vi "On Open Document.vi"(0 "PDF Report IN":T23(xcontrol), 11 "error in (no error)":errorcluster) -> (4 "PDF Report OUT":T23(xcontrol), 15 "error out":errorcluster)   [LabVIEW 2013]
doc: "Developed by Jean-Marc Simard\nCopyright © 2010, Exaprom Inc.\nAll rights reserved.\nLicense: BSD\n\nWith iTextSharp 4.1.6 (http://itextsharp.sourceforge.net)\nunder Mozilla Public License Version 1.1\n(http://www.mozilla.org/MPL/MPL-1.1.html)"
uses:
  C:/Users/MaxCorp/Documents/GitHub/TopView/DLL/itextsharp.dll
  DLL/itextsharp.dll
  Controls/PDF Report Xcontrol/PDF Report.xctl
  Controls/Font size.ctl
  Controls/Font color.ctl
  Controls/Font cluster.ctl
  Controls/Header footer horiz alignment.ctl
  <userlib>/Exaprom PDF/Controls/Watermark Page Position.ctl
  Controls/Watermark cluster.ctl
panel:
  out "Font OUT":T1={"Name"="Helvetica", "Size"=12.0, "Color"=0, "Style"={"Bold"=FALSE, "Italic"=FALSE, "Underline"=FALSE, "Strikeout"=FALSE}}
  in  "Font IN":T1={"Name"="Helvetica", "Size"=12.0, "Color"=0, "Style"={"Bold"=FALSE, "Italic"=FALSE, "Underline"=FALSE, "Strikeout"=FALSE}}
  in  "input cluster":T4={"Show? (F)"=FALSE, "Watermark type"=enum."Text", "Opacity (%)"=0.0, "Alignment"=enum."Center", "Rotate(°)"=0.0, "Watermark"=enum."Absolute", "X (mm)"=5.0, "Y (mm)"=30.0, "Text"="JMS", "Font"={"Name"="", "Size"=12.0, "Color"=0, "Style"={"Bold"=FALSE, "Italic"=FALSE, "Underline"=FALSE, "Strikeout"=FALSE}}, "Image path"=path "", "Image (%)"=100.0}
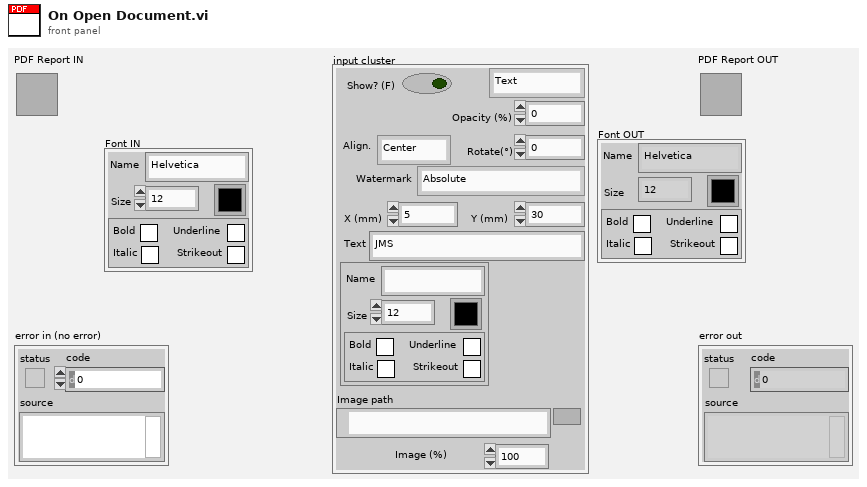
[diagram p1: front panel]
types:
  T1 = typedef "Font cluster.ctl" = cluster{"Name":string, "Size":T2, "Color":T3, "Style":cluster{"Bold":bool, "Italic":bool, "Underline":bool, "Strikeout":bool}}
  T2 = typedef "Font size.ctl" = sgl
  T3 = typedef "Font color.ctl" = u32
  T4 = typedef "Watermark cluster.ctl" = cluster{"Show? (F)":bool, "Watermark type":enum16{"Text", "Text auto", "Image"}, "Opacity (%)":sgl, "Alignment":T5, "Rotate(°)":sgl, "Watermark":T6, "X (mm)":sgl, "Y (mm)":sgl, "Text":string, "Font":T1, "Image path":path, "Image (%)":sgl}
  T5 = typedef "Header footer horiz alignment.ctl" = enum16{"Left", "Center", "Right"}
  T6 = typedef "Watermark Page Position.ctl" = enum16{"Absolute", "Center on page", "Center on text section"}
  T7 = typedef "Unit.ctl" = enum16{"inch", "mm"}
  T8 = typedef "Paragraphe cluster.ctl" = cluster{" Aligment":T9, "Line spacing":T10}
  T9 = typedef "Texte alignement.ctl" = enum16{"Select", "CENTER", "JUSTIFY", "LEFT", "RIGHT"}
  T10 = typedef "Line spacing.ctl" = enum16{"Select", "1.0", "1.5", "2.0"}
  T11 = typedef "Page dimensions.ctl" = cluster{"Start at page":i32, "Orientation":T12, "widht":sgl, "height":sgl, "Margin left":sgl, "Margin right":sgl, "Margin top":sgl, "Margin bottom":sgl}
  T12 = typedef "Page Orientation.ctl" = enum16{"Portrait", "Landscape"}
  T13 = typedef "Image or Table Caption.ctl" = cluster{"Caption":string, "Separator":string, "Position":enum16{"Above", "Below"}}
  T14 = typedef "Header Footer [ ].ctl" = T15[]
  T15 = typedef "Header Footer cluster.ctl" = cluster{"Start page":i32, "Type":T16, "Alignment":T5, "Vertical Alignement":T17, "Image (%)":sgl, "Page #":T18, "Text":string, "Path":string, "Font":T1, "Font refnum":refnum<k24>, "Line":cluster{"Line":T19, "Thickness (points)":sgl, "Colour":T3}}
  T16 = typedef "Header Footer Type.ctl" = enum16{"Select", "Text", "Text + hyperlink", "Page number", "Image", "Image + hyperlink"}
  T17 = typedef "Cell Vertical alignment.ctl" = enum16{"TOP", "MIDDLE", "BOTTOM"}
  T18 = typedef "Page number.ctl" = cluster{"Text 1":string, "Text 2":string, "Text 3":string}
  T19 = typedef "Header Footer Line.ctl" = enum16{"No line", "Horizontal line"}
  T20 = typedef "Watermark cluster2.ctl" = cluster{"Show? (F)":bool, "Type":enum16{"Image", "Text"}, "Opacity (%)":sgl, "Rotate(°)":sgl, "Position":cluster{"Position":T21, "X":sgl, "Y":sgl}, "Image path":path, "Scaled(%)":sgl, "Image refnum":refnum<k24>, "Text":string, "Font":cluster{"Name":string, "Size":T2, "Color":T3}, "Font refnum":refnum<k24>, "Alignment":T5, "Automatic":bool}
  T21 = typedef "Watermark Position.ctl" = enum16{"Absolute", "Center (page)", "Center (text section)"}
  T22 = typedef "System Fonts.ctl" = cluster{"Font name [ ]":string[], "Font and file names [ ]":cluster{"Font name":string, "File name":string}[]}
  T23 = cluster{"Document":refnum<k24>, "Writer":refnum<k24>, "Default Font":refnum<k24>, "Default Font cluster":T1, "Path":path, "Unit (default = mm)":T7, "Paragraphe cluster":T8, "Pages dimensions [ ]":T11[], "Captions":cluster{"Image":T13, "Image counter":u16, "Table":T13, "Table counter":u16, "Font":T1}, "Header":T14, "Footer":T14, "Watermark ":T20, "Actual VI name":string, "System Fonts":T22}
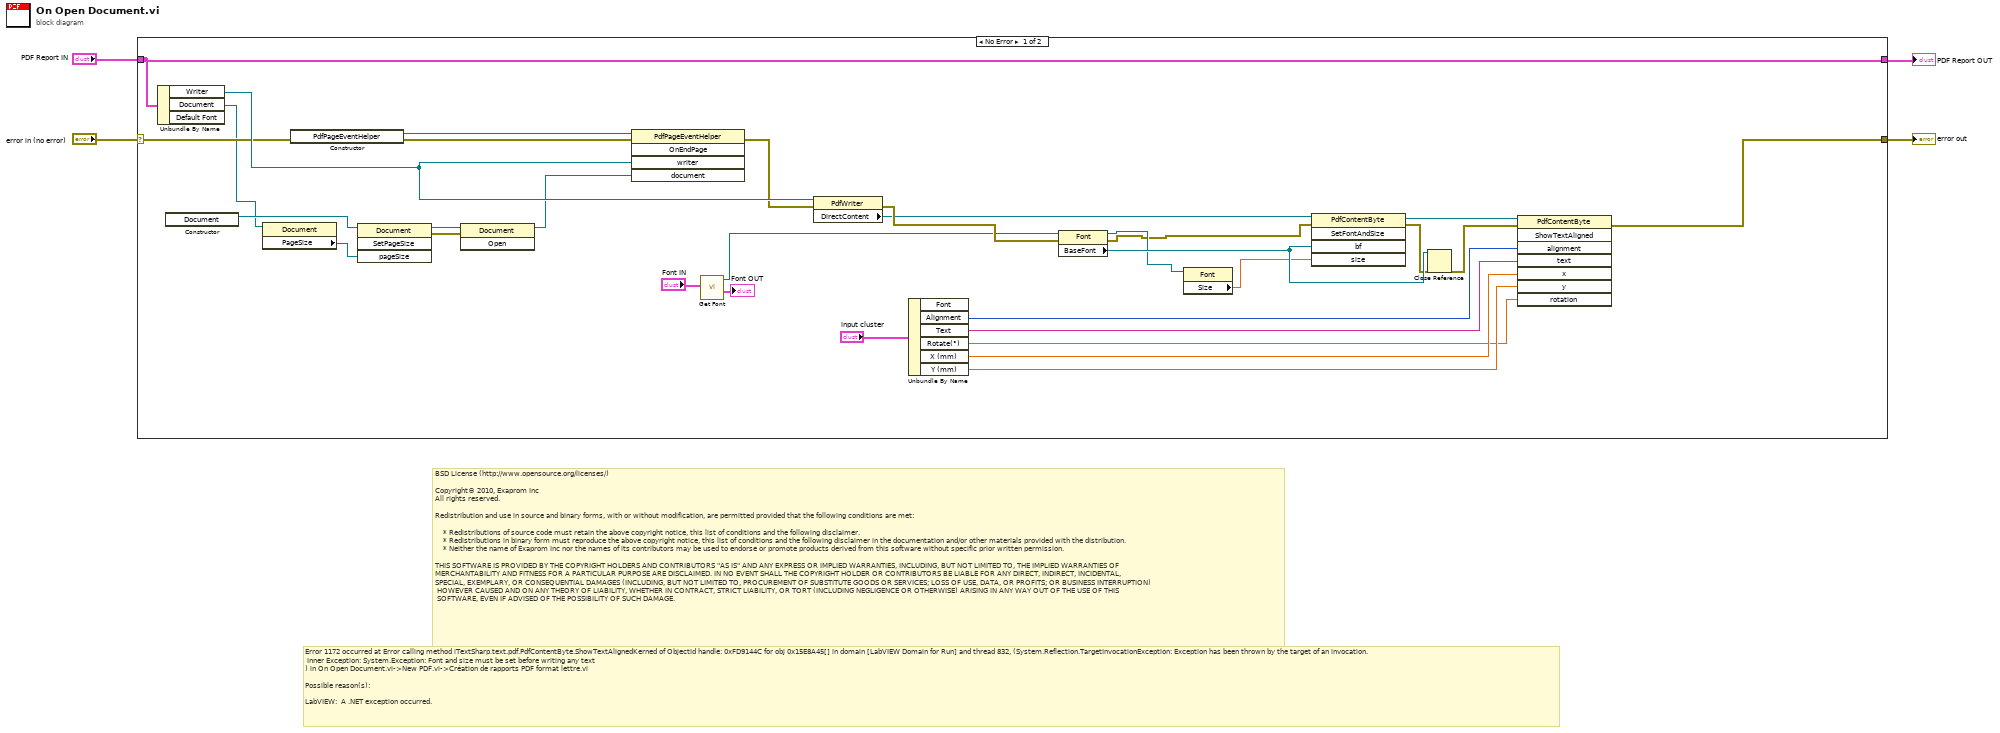
[diagram p0: block diagram]
diagram:
  # "Error 1172 occurred at Error calling method iTextSharp.text.pdf.PdfContentByte.ShowTextAlignedKerned of ObjectId handle: 0xFD9144C for obj 0x15E8A45[] in domain [LabVIEW Domain for Run] and thread 832, (System.Reflection.TargetInvocationException: Exception has been thrown by the target of an invocation.\n\tInner Exception: System.Exception: Font and size must be set before writing any text\n) in On Open Document.vi->New PDF.vi->Création de rapports PDF format lettre.vi\n\nPossible reason(s):\n\nLabVIEW:  A .NET exception occurred."
  # "BSD License (http://www.opensource.org/licenses/)\n\nCopyright© 2010, Exaprom Inc\nAll rights reserved.\n\nRedistribution and use in source and binary forms, with or without modification, are permitted provided that the following conditions are met:\n\n    * Redistributions of source code must retain the above copyright notice, this list of conditions and the following disclaimer.\n    * Redistributions in binary form must reproduce the above copyright notice, this list of conditions and the following disclaimer in the documentation and/or other materials provided with the distribution.\n    * Neither the name of Exaprom Inc nor the names of its contributors may be used to endorse or promote products derived from this software without specific prior written permission.\n\nTHIS SOFTWARE IS PROVIDED BY THE COPYRIGHT HOLDERS AND CONTRIBUTORS \"AS IS\" AND ANY EXPRESS OR IMPLIED WARRANTIES, INCLUDING, BUT NOT LIMITED TO, THE IMPLIED WARRANTIES OF \nMERCHANTABILITY AND FITNESS FOR A PARTICULAR PURPOSE ARE DISCLAIMED. IN NO EVENT SHALL THE COPYRIGHT HOLDER OR CONTRIBUTORS BE LIABLE FOR ANY DIRECT, INDIRECT, INCIDENTAL,\nSPECIAL, EXEMPLARY, OR CONSEQUENTIAL DAMAGES (INCLUDING, BUT NOT LIMITED TO, PROCUREMENT OF SUBSTITUTE GOODS OR SERVICES; LOSS OF USE, DATA, OR PROFITS; OR BUSINESS INTERRUPTION)\n HOWEVER CAUSED AND ON ANY THEORY OF LIABILITY, WHETHER IN CONTRACT, STRICT LIABILITY, OR TORT (INCLUDING NEGLIGENCE OR OTHERWISE) ARISING IN ANY WAY OUT OF THE USE OF THIS\n SOFTWARE, EVEN IF ADVISED OF THE POSSIBILITY OF SUCH DAMAGE."
  n1 = case shown="No Error" "error in (no error)" {
    selector: "error in (no error)" -> [w31 w37]
    tunnel: "PDF Report IN" -> [w35 w36]
    tunnel: [w35 w36] -> w3
    tunnel: [w18 w37] -> w2
    frame No Error {
      n2 = Unbundle By Name(w35) -> ("Writer"=w34:refnum<k24>, "Document"=w7:refnum<k24>)  [unwired: 1 out]
      n3 = constructor class="Document"() -> (reference out=w11:refnum<k24>)  [unwired: 3 in, 2 out]
      n4 = property class="Document"(reference=w7) -> ("PageSize"=w10:refnum<k24>)  [unwired: 1 in, 2 out]
      n5 = constructor class="PdfPageEventHelper"(error in=w31) -> (reference out=w30:refnum<k24>, error out=w33:errorcluster)  [unwired: 2 in, 1 out]
      n6 = invoke class="Document" method="SetPageSize"(reference=w11, "pageSize"=w10) -> (reference out=w9:refnum<k24>, error out=w8:errorcluster)  [unwired: 2 in, 2 out]
      n7 = invoke class="Document" method="Open"(reference=w9, error in=w8) -> (reference out=w6:refnum<k24>)  [unwired: 1 in, 2 out]
      n8 = invoke class="PdfPageEventHelper" method="OnEndPage"(reference=w30, error in=w33, "writer"=w34, "document"=w6) -> (error out=w32:errorcluster)  [unwired: 1 in, 4 out]
      n9 = call "Get Font.vi"("Font IN"="Font IN") -> ("Font OUT"=→"Font OUT":T1, "Font"=w14:refnum<k24>)  [unwired: 2 in, 7 out]
      n10 = property class="PdfWriter"(reference=w34, error in=w32) -> (error out=w20:errorcluster, "DirectContent"=w12:refnum<k24>)  [unwired: 1 out]
      n11 = Unbundle By Name("input cluster") -> ("Alignment"=w26:T5, "Text"=w27:string, "Rotate(°)"=w21:sgl, "X (mm)"=w22:sgl, "Y (mm)"=w23:sgl)  [unwired: 1 out]
      n12 = property class="Font"(reference=w14, error in=w20) -> (reference out=w17:refnum<k24>, error out=w13:errorcluster, "BaseFont"=w28:refnum<k24>)
      n13 = property class="Font"(reference=w17) -> ("Size"=w16:sgl)  [unwired: 1 in, 2 out]
      n14 = invoke class="PdfContentByte" method="SetFontAndSize"(reference=w12, error in=w13, "bf"=w28, "size"=w16) -> (reference out=w29:refnum<k24>, error out=w24:errorcluster)  [unwired: 1 in, 3 out]
      n15 = Close Reference(reference=w28, error in (no error)=w24) -> (error out=w25:errorcluster)
      n16 = invoke class="PdfContentByte" method="ShowTextAligned"(reference=w29, error in=w25, "alignment"=w26, "text"=w27, "x"=w22, "y"=w23, "rotation"=w21) -> (error out=w18:errorcluster)  [unwired: 1 in, 7 out]
    }
    frame Error {
    }
  }
  "PDF Report OUT" <- w3
  "error out" <- w2
